vi "Check for Critical NTC.vi"(11 "NTCs":sgl[](array[numeric])) -> (3 "Critical NTC":bool)   [LabVIEW 2025]
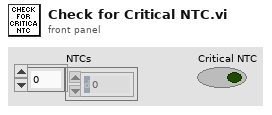
[diagram p1: front panel]
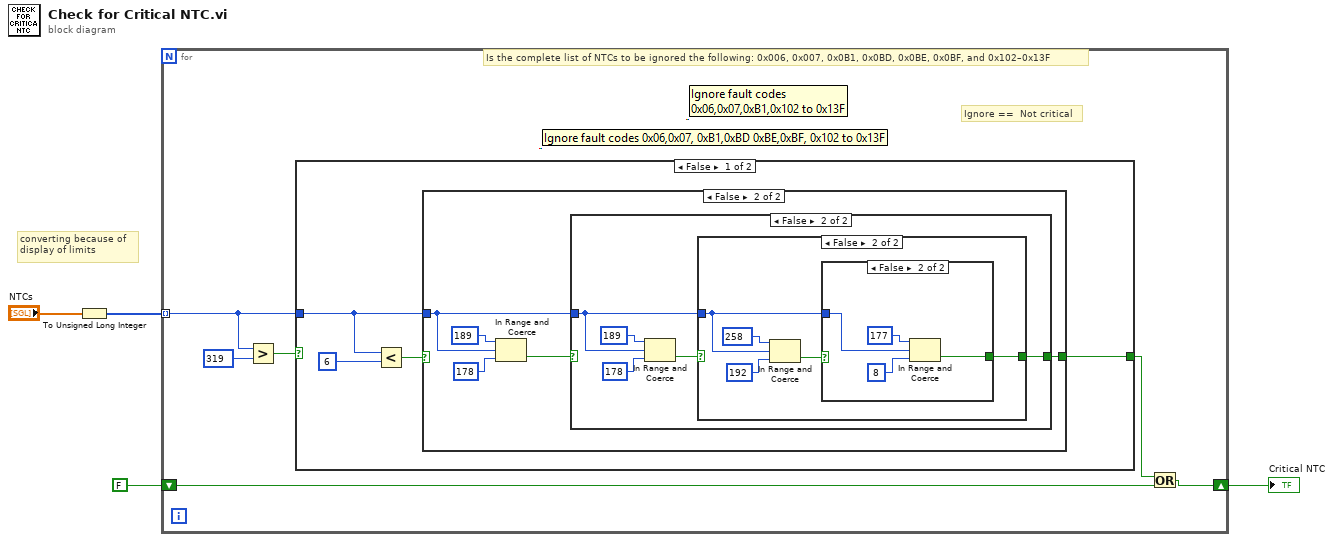
[diagram p0: block diagram]
diagram:
  # "converting because of\ndisplay of limits"
  n1 = To Unsigned Long Integer(number="NTCs") -> (unsigned 32bit integer=w1:u32[])
  n2 = for {
    tunnel: w1 -> [w8] mode=indexing
    shift-right: [w5] -> w4
    shift-left: FALSE -> [w6]
    # "Ignore ==  Not critical"
    # "Is the complete list of NTCs to be ignored the following: 0x006, 0x007, 0x0B1, 0x0BD, 0x0BE, 0x0BF, and 0x102–0x13F"
    n3 = Greater?(x=w8, y=u32 319) -> (0:w9:bool)
    n4 = case shown="False" w9 {
      selector: w9 -> [_ w38]
      tunnel: w8 -> [w11 _]
      tunnel: [w14 w38] -> w7
      frame False {
        n5 = Less?(x=w11, y=u32 6) -> (x < y?=w12:bool)
        n6 = case shown="False" w12 {
          selector: w12 -> [w15 _]
          tunnel: w11 -> [_ w17]
          tunnel: [w15 w16] -> w14
          frame True {
          }
          frame False {
            n7 = In Range and Coerce(upper limit=u32 189 ("y"), x=w17, lower limit=u32 178 ("y")) -> (In Range?=w18:bool)  [unwired: 1 out]
            n8 = case shown="False" w18 {
              selector: w18 -> [w21 _]
              tunnel: w17 -> [_ w23]
              tunnel: [w21 w22] -> w16
              frame True {
              }
              frame False {
                n9 = In Range and Coerce(upper limit=u32 189 ("y"), x=w23, lower limit=u32 178 ("y")) -> (In Range?=w24:bool)  [unwired: 1 out]
                n10 = case shown="False" w24 {
                  selector: w24 -> [w27 _]
                  tunnel: w23 -> [_ w29]
                  tunnel: [w27 w28] -> w22
                  frame True {
                  }
                  frame False {
                    n11 = In Range and Coerce(upper limit=u32 258 ("y"), x=w29, lower limit=u32 192 ("y")) -> (In Range?=w30:bool)  [unwired: 1 out]
                    n12 = case shown="False" w30 {
                      selector: w30 -> [w33 _]
                      tunnel: w29 -> [_ w35]
                      tunnel: [w33 w34] -> w28
                      frame True {
                      }
                      frame False {
                        n13 = In Range and Coerce(upper limit=u32 177 ("y"), x=w35, lower limit=u32 8 ("y")) -> (In Range?=w34:bool)  [unwired: 1 out]
                      }
                    }
                  }
                }
              }
            }
          }
        }
      }
      frame True {
      }
    }
    n14 = Or(x=w7, y=w6) -> (x .or. y?=w5:bool)
  }
  "Critical NTC" <- w4
